vi "Wilcoxon Signed-Rank Test (paired samples).vi"(6 "alternative hypothesis":i32(ring) items=["mean(x) != mean(y)"=0, "mean(x) > mean(y)"=1, "mean(x) < mean(y)"=-1], 9 "significance level":dbl=0.05, 10 "sample set y":dbl[](array[numeric]), 11 "sample set x":dbl[](array[numeric])) -> (0 "error":i32, 2 "p value":dbl=0.05 format="%.6g", 3 "reject null hypothesis":bool)   [LabVIEW 2014, in "NI_Gmath.lvlib"]
doc: "Tests hypotheses about the <B>mean</B> of populations whose distributions are continuous and symmetric but not necessarily normal. You must manually select the polymorphic instance to use."
uses:
  NI_Gmath.lvlib
panel:
  # "Wilcoxon Signed-Rank Test"
  # "null hypothesis\nmean(pop) = mean"
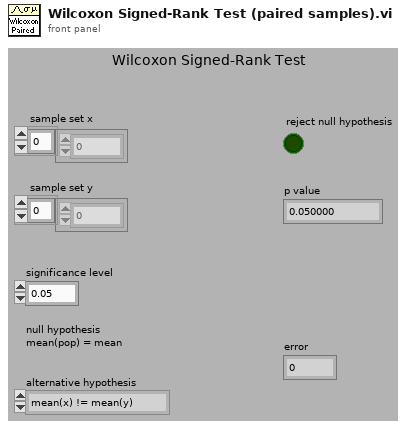
[diagram p1: front panel]
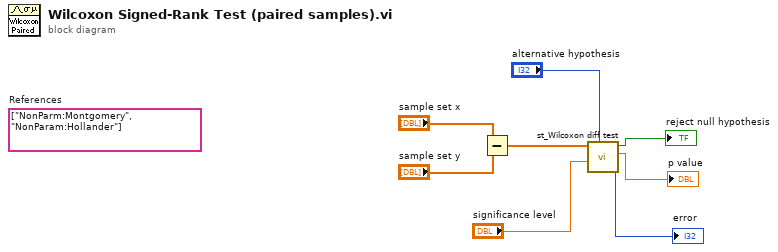
[diagram p0: block diagram]
diagram:
  (unwired) string[] ["NonParm:Montgomery", "NonParam:Hollander"]  # References
  n1 = Subtract(x="sample set x", y="sample set y") -> (x-y=w3:dbl[])
  n2 = call "st_Wilcoxon diff test.vi"("alternative hypothesis"="alternative hypothesis", "significance level"="significance level", "Xi - Yi"=w3) -> ("error"=→"error":i32, "p value"=→"p value":dbl, "reject the null hypothesis"=→"reject null hypothesis":bool)  [unwired: 6 in]
